vi "Temp to data array.vi"(11 "Temperature":dbl) -> (3 "Data":u8[](array[numeric]))   [LabVIEW 2018, in "EF20.lvlib" / "EF20.lvclass"]
uses:
  EF20.lvclass
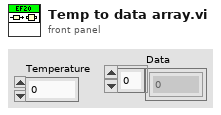
[diagram p1: front panel]
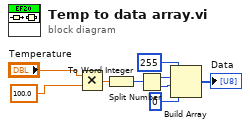
[diagram p0: block diagram]
diagram:
  n1 = Multiply(x="Temperature", y=100.0) -> (x*y=w9:dbl)
  n2 = To Word Integer(number=w9) -> (16bit integer=w8:i16)
  n3 = Split Number(x=w8) -> (hi(x)=w7:u8, lo(x)=w6:u8)
  n4 = Build Array(u8 255 ("element"), w7, w6, u8 0 ("element")) -> (→"Data":u8[])
